vi "LeftPanel.vi"(3 "Left Panel":T3 {"Electrode 16"."Magnitude" format="%4.2f"; "Electrode 15"."Magnitude" format="%4.2f"; "Electrode 14"."Magnitude" format="%4.2f"; "Electrode 13"."Magnitude" format="%4.2f"; "Electrode 12"."Magnitude" format="%4.2f"; "Electrode 11"."Magnitude" format="%4.2f"; "Electrode 10"."Magnitude" format="%4.2f"; "Electrode 9"."Magnitude" format="%4.2f"; "Electrode 8"."Magnitude" format="%4.2f"; "Electrode 7"."Magnitude" format="%4.2f"; "Electrode 6"."Magnitude" format="%4.2f"; "Electrode 5"."Magnitude" format="%4.2f"; "Electrode 4"."Magnitude" format="%4.2f"; "Electrode 3"."Magnitude" format="%4.2f"; "Electrode 2"."Magnitude" format="%4.2f"; "Electrode"."Magnitude" format="%4.2f"}, 10 "Seqn in":refnum<class "Sequence.lvclass">, 11 "LP Refnum":refnum<vi>) -> ()   [LabVIEW 2012]
uses:
  UserControl/LeftPanel.ctl
  UserControl/ElectdPanel.ctl
  UserControl/ElectdTerminal.ctl
  Sequence.lvclass
  Cohort.lvclass
  StimulCtrls.lvlib
panel:
  out "Electrode":T1 {"Magnitude" format="%4.2f"}
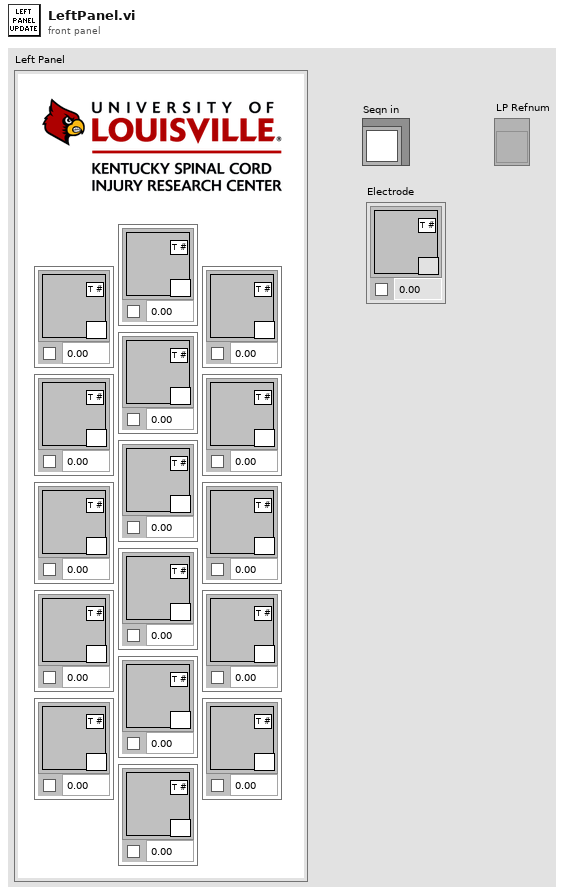
[diagram p1: front panel]
types:
  T1 = typedef "StimulCtrls.lvlib/ElectdPanel.ctl" = cluster{"Group #":string, "T #":T2, "Magnitude":sgl, "check":bool}
  T2 = typedef "StimulCtrls.lvlib/ElectdTerminal.ctl" = u8
  T3 = typedef "StimulCtrls.lvlib/LeftPanel.ctl" = cluster{"Electrode":T1, "Electrode 2":T1, "Electrode 3":T1, "Electrode 4":T1, "Electrode 5":T1, "Electrode 6":T1, "Electrode 7":T1, "Electrode 8":T1, "Electrode 9":T1, "Electrode 10":T1, "Electrode 11":T1, "Electrode 12":T1, "Electrode 13":T1, "Electrode 14":T1, "Electrode 15":T1, "Electrode 16":T1}
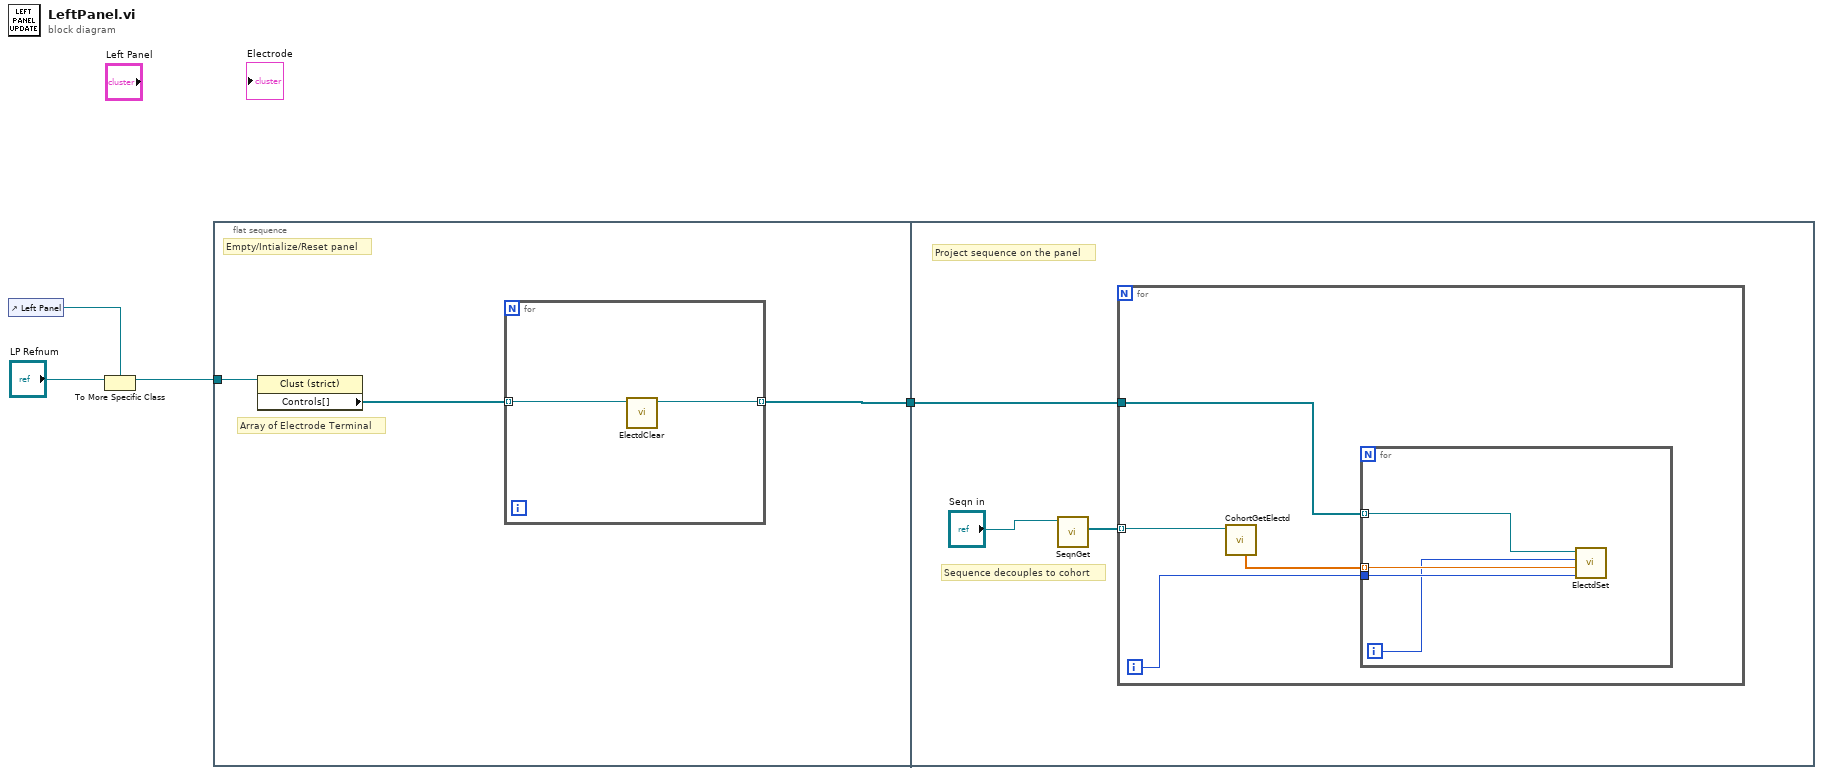
[diagram p0: block diagram]
diagram:
  n1 = control-ref of="Left Panel"() -> (w1:refnum<vi>)
  n2 = To More Specific Class(target class=w1, reference="LP Refnum") -> (specific class reference=w3:refnum<vi>)  [unwired: 1 in, 1 out]
  n3 = flat-sequence {
    tunnel: w3 -> [w7]
    tunnel: [w5] -> w4
    tunnel: w4 -> [w10]
    frame #0 {
      # "Empty/Intialize/Reset panel"
      # "Array of Electrode Terminal"
      n4 = property class="Clust (strict)"(reference=w7) -> ("Controls[]"=w6:refnum<vi>[])  [unwired: 1 in, 2 out]
      n5 = for {
        tunnel: w6 -> [w8] mode=indexing
        tunnel: [w9] -> w5 mode=indexing
        n6 = call "ElectdClear.vi"("Electd in"=w8) -> ("Electd out"=w9:refnum<vi>)  [unwired: 10 in]
      }
    }
    frame #1 {
      # "Sequence decouples to cohort"
      # "Project sequence on the panel"
      n7 = call-dynamic "SeqnGet.vi"("Sequence in"="Seqn in") -> ("Cohorts"=w11:refnum<class "Cohort.lvclass">[])  [unwired: 8 in, 2 out]
      n8 = for {
        tunnel: w11 -> [w16] mode=indexing
        tunnel: w10 -> [w13]
        i -> [w14]
        n9 = call-dynamic "CohortGetElectd.vi"("Cohort in"=w16) -> ("Amplitude"=w15:sgl[])  [unwired: 6 in, 4 out]
        n10 = for {
          tunnel: w15 -> [w20] mode=indexing
          tunnel: w14 -> [w19]
          tunnel: w13 -> [w17] mode=indexing
          i -> [w18]
          n11 = call "ElectdSet.vi"("Group #"=w19, "Amplitude"=w20, "Index"=w18, "Electd Panel in"=w17) -> ()  [unwired: 7 in, 1 out]
        }
      }
    }
  }
